vi "NI 9237_Config.vi"(8 "error in":errorcluster, 11 "task in":refnum<k21>) -> (0 "error out":errorcluster, 3 "task out":refnum<k21>)   [LabVIEW 2022 SP3]
uses:
  <vilib>/DAQmx/create/channels.llb/DAQmx Create Channel (AI-Force-Bridge-Two-Point-Linear).vi
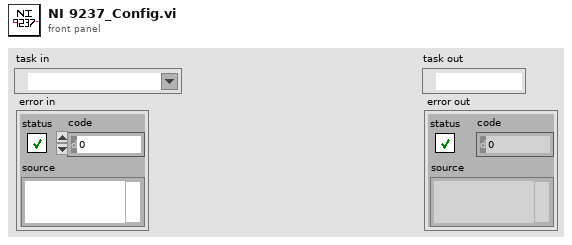
[diagram p1: front panel]
types:
  T1 = cluster{"bridge configuration":i32, "voltage excitation source":i32, "voltage excitation value":dbl, "nominal bridge resistance":dbl}
  T2 = cluster{"first electrical value":dbl, "second electrical value":dbl, "electrical units":i32, "first physical value":dbl, "second physical value":dbl, "physical units":i32}
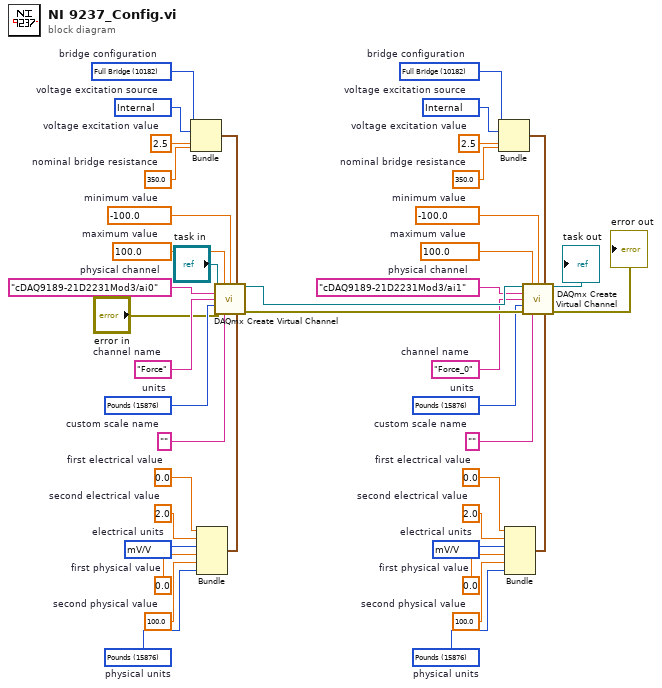
[diagram p0: block diagram]
diagram:
  w5 = 15876 items=["Newtons"=15875, "Pounds"=15876, "kgf"=15877]  # physical units
  w11 = 0.0  # first electrical value
  w10 = 2.0  # second electrical value
  w9 = 15897 items=["V/V"=15896, "mV/V"=15897]  # electrical units
  w8 = 0.0  # first physical value
  w7 = 100.0  # second physical value
  w13 = 350.0  # nominal bridge resistance
  w14 = 2.5  # voltage excitation value
  w15 = 10200 items=["Internal"=10200, "External"=10167]  # voltage excitation source
  w16 = 10182 items=["Full Bridge"=10182, "Half Bridge"=10187, "Quarter Bridge"=10270]  # bridge configuration
  w17 = 15876 items=["Newtons"=15875, "Pounds"=15876, "kgf"=15877, "From Custom Scale"=10065]  # units
  w18 = "Force_0"  # channel name
  w19 = ""  # custom scale name
  w20 = -100.0  # minimum value
  w21 = 100.0  # maximum value
  w22 = "cDAQ9189-21D2231Mod3/ai1"  # physical channel
  w24 = 15876 items=["Newtons"=15875, "Pounds"=15876, "kgf"=15877]  # physical units
  w30 = 0.0  # first electrical value
  w29 = 2.0  # second electrical value
  w28 = 15897 items=["V/V"=15896, "mV/V"=15897]  # electrical units
  w27 = 0.0  # first physical value
  w26 = 100.0  # second physical value
  w32 = 350.0  # nominal bridge resistance
  w33 = 2.5  # voltage excitation value
  w34 = 10200 items=["Internal"=10200, "External"=10167]  # voltage excitation source
  w35 = 10182 items=["Full Bridge"=10182, "Half Bridge"=10187, "Quarter Bridge"=10270]  # bridge configuration
  w36 = 15876 items=["Newtons"=15875, "Pounds"=15876, "kgf"=15877, "From Custom Scale"=10065]  # units
  w37 = "Force"  # channel name
  w39 = ""  # custom scale name
  w40 = -100.0  # minimum value
  w41 = 100.0  # maximum value
  w42 = "cDAQ9189-21D2231Mod3/ai0"  # physical channel
  n1 = Bundle("bridge configuration"=w35, "voltage excitation source"=w34, "voltage excitation value"=w33, "nominal bridge resistance"=w32) -> (w31:T1)  [unwired: 1 in]
  n2 = Bundle("first electrical value"=w30, "second electrical value"=w29, "electrical units"=w28, "first physical value"=w27, "second physical value"=w26, "physical units"=w24) -> (w25:T2)  [unwired: 1 in]
  n3 = call-poly <vilib>:"DAQmx Create Virtual Channel.vi"("task in"="task in", "maximum value"=w41, "minimum value"=w40, "bridge information"=w31, "physical channels"=w42, "name to assign"=w37, "units"=w36, "error in"="error in", "custom scale name"=w39, "scaling information"=w25) -> ("task out"=w23:refnum<k21>, "error out"=w38:errorcluster)  [unwired: 4 in]
  n4 = Bundle("bridge configuration"=w16, "voltage excitation source"=w15, "voltage excitation value"=w14, "nominal bridge resistance"=w13) -> (w12:T1)  [unwired: 1 in]
  n5 = Bundle("first electrical value"=w11, "second electrical value"=w10, "electrical units"=w9, "first physical value"=w8, "second physical value"=w7, "physical units"=w5) -> (w6:T2)  [unwired: 1 in]
  n6 = call-poly <vilib>:"DAQmx Create Virtual Channel.vi"("task in"=w23, "maximum value"=w21, "minimum value"=w20, "bridge information"=w12, "physical channels"=w22, "name to assign"=w18, "units"=w17, "error in"=w38, "custom scale name"=w19, "scaling information"=w6) -> ("task out"=→"task out":refnum<k21>, "error out"=→"error out":errorcluster)  [unwired: 4 in]
